vi "Get Devs and Channels.vi"(8 "error in (no error)":errorcluster, 11 "DAQmx Sequencer in":refnum<class "DAQmx Sequencer.lvclass">) -> (0 "error out":errorcluster, 3 "DAQmx Sequencer out":refnum<class "DAQmx Sequencer.lvclass">)   [LabVIEW 2015, in "Sequencer.lvlib"]
uses:
  Sequencer/Sequencer.lvlib
  <resource>/objmgr/daqmx.rc
  Sequencer/Sequencer/Daq Channel Info.ctl
  Sequencer/Sequencer/Sequencer.lvclass
  DAQmx Sequencer.lvclass
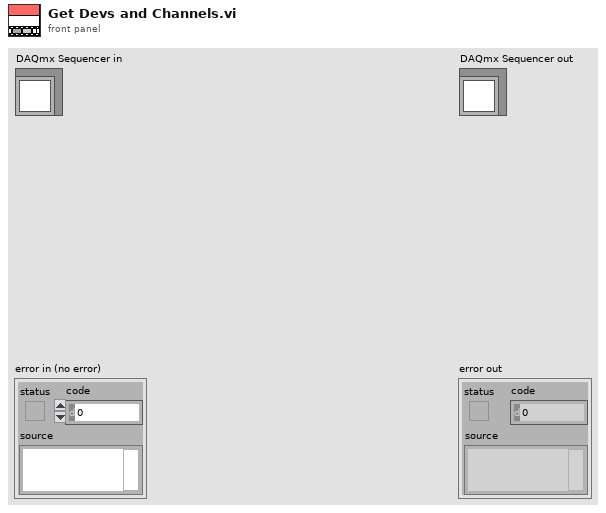
[diagram p1: front panel]
types:
  T1 = typedef "Sequencer.lvlib/Sequencer.lvclass/Daq Channel Info.ctl" = cluster{"DevNames":tag[], "AO.PhysicalChans":tag[][], "DO.Lines":tag[][], "AI.PhysicalChans":tag[][]}
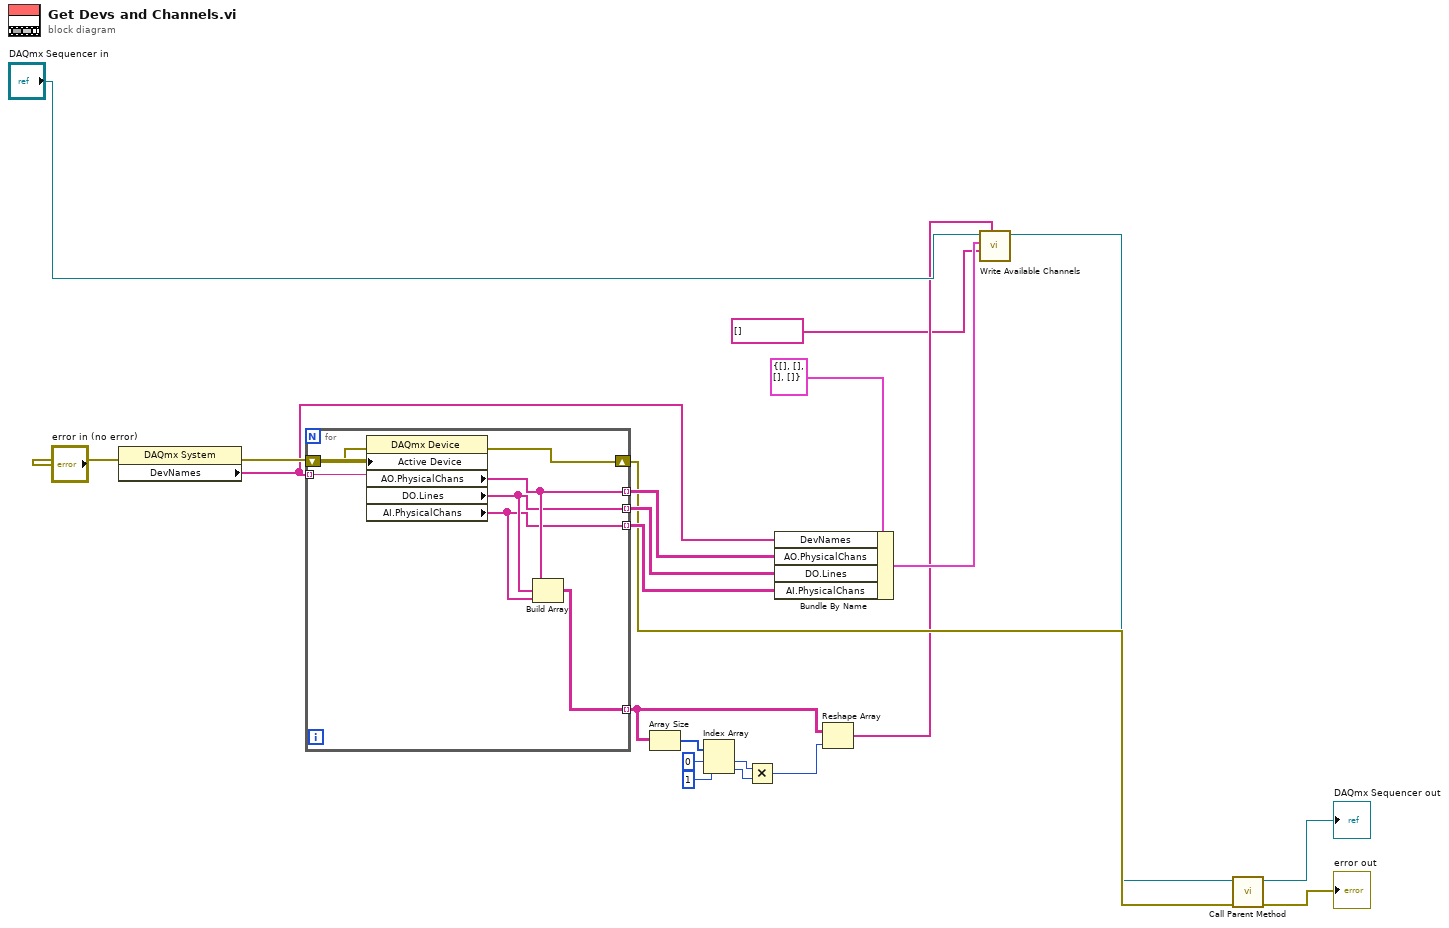
[diagram p0: block diagram]
diagram:
  n1 = property class="DAQmx System"(error in="error in (no error)") -> (error out=w20:errorcluster, "DevNames"=w19:tag[])  [unwired: 1 in, 1 out]
  n2 = for {
    tunnel: w19 -> [w29] mode=indexing
    tunnel: [w26] -> w16 mode=indexing
    tunnel: [w25] -> w17 mode=indexing
    tunnel: [w24] -> w18 mode=indexing
    shift-right: [w27] -> w7
    shift-left: w20 -> [w28]
    tunnel: [w23] -> w10 mode=indexing
    n3 = property class="DAQmx Device"(error in=w28, "Active Device"=w29) -> (error out=w27:errorcluster, "AO.PhysicalChans"=w26:tag[], "DO.Lines"=w25:tag[], "AI.PhysicalChans"=w24:tag[])  [unwired: 1 in, 1 out]
    n4 = Build Array(w26, w25, w24) -> (w23:tag[][])
  }
  n5 = Array Size(array=w10) -> (size(s)=w15:i32[])
  n6 = Index Array(array=w15, index #1=0 ("index"), index #2=1 ("index")) -> (element #1=w12:i32, element #2=w11:i32)
  n7 = Multiply(x=w12, y=w11) -> (x*y=w9:i32)
  n8 = Bundle By Name(cluster=T1 {"DevNames"=[], "AO.PhysicalChans"=[], "DO.Lines"=[], "AI.PhysicalChans"=[]} ("DAQ Channel Info"), "DevNames"=w19, "AO.PhysicalChans"=w16, "DO.Lines"=w17, "AI.PhysicalChans"=w18) -> (w3:T1)
  n9 = Reshape Array(w10, w9) -> (w2:tag[])
  n10 = call "Write Available Channels.vi"("All Daq Channels"=w2, "Used DAQChannels"=tag[] [], "DAQ Channel Info"=w3, "Sequencer in"="DAQmx Sequencer in") -> ("Sequencer out"=w4:refnum<class "DAQmx Sequencer.lvclass">)  [unwired: 6 in, 1 out]
  n11 = call-parent "Call Parent Method"("error in (no error)"=w7, "Sequencer in"=w4) -> ("error out"=→"error out":errorcluster, "Sequencer out"=→"DAQmx Sequencer out":refnum<class "DAQmx Sequencer.lvclass">)  [unwired: 8 in]
